vi "Teleop.vi"(0 "Call Context":T10) -> (6 "SubState 3":T1, 8 "SubState 4":T1, 9 "SubState 5":T9, 11 "Loop 3 Data":T5, 13 "Loop 4 Data":T4, 14 "SubState 0":T1=enum."driver control", 15 "Loop 1 Data":T7, 16 "Loop 0 Data":T8, 17 "SubState 1":T1, 18 "Loop 2 Data":T6, 19 "SubState 2":T1)   [LabVIEW 2013]
uses:
  typedefs/subStates.ctl
  <vilib>/Rock Robotics/WPI/DriverStation/WPI_DriverStationDerivedRobotMode.ctl
  typedefs/singleUseSubstate.ctl
  typedefs/Loop Datatypes/Loop 0 Datatype.ctl
  typedefs/Loop Datatypes/Loop 1 Datatype.ctl
  typedefs/Loop Datatypes/Loop 2 Datatype.ctl
  typedefs/Loop Datatypes/Loop 3 Datatype.ctl
  typedefs/Loop Datatypes/Loop 4 Datatype.ctl
  <vilib>/Rock Robotics/WPI/Joystick/WPI_JoystickDevRef.ctl
  <vilib>/Rock Robotics/WPI/Joystick/WPI_JoystickDeviceEnum.ctl
  typedefs/fg_typedef.ctl
  typedefs/vision enable.ctl
  <vilib>/Rock Robotics/WPI/Joystick/WPI_JoystickGetSetRefNum.vi
panel:
  out "prev lock state":T1
  out "JS3":T2
  out "Drive to DC":bool
  out "JS1":T2
  out "JS2":T2
  out "Exit Value":i32=-1
  # "Loop Data and Substates"
  # "Latch Loop"
  # "Drive Loop"
  # "Shooter Pneumatics Loop"
  # "Pickup/Passing Belts Loop"
  # "Pickup Arm Loop"
  # "Shifter Loop"
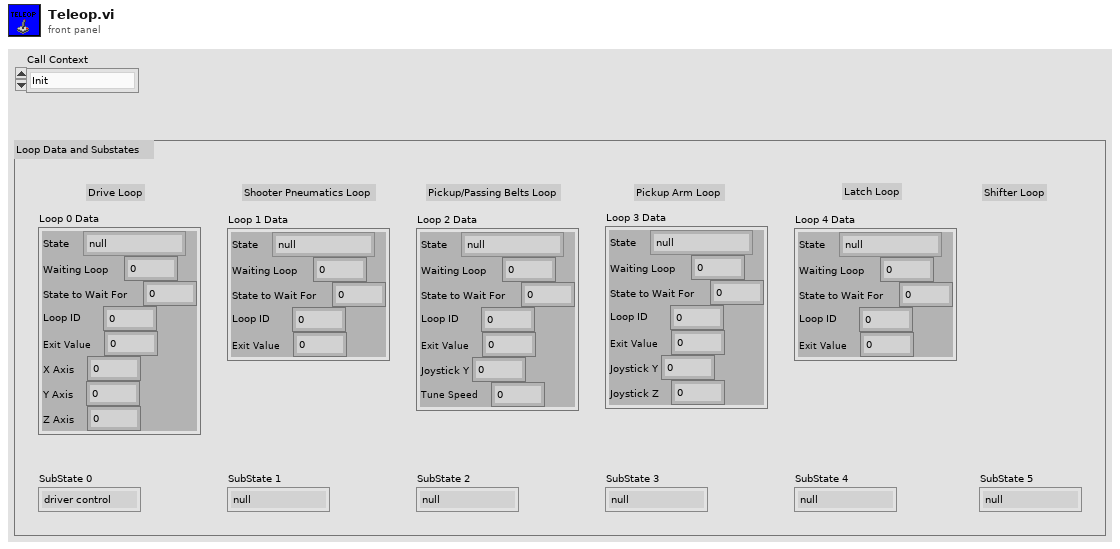
[diagram p1: front panel]
types:
  T1 = typedef "subStates.ctl" = enum16{"null", "wait", "driver control", "auto", "manual override", "hold position", "rotate", "pickup", "pass", "load", "goto shoot", "shoot", "cancel", "end"}
  T2 = typedef "WPI_JoystickDevRef.ctl" = cluster{"Device":T3}
  T3 = typedef "WPI_JoystickDeviceEnum.ctl" = enum16{"USB 1", "USB 2", "USB 3", "USB 4", "Kinect 1", "Kinect 2"}
  T4 = typedef "Loop 4 Datatype.ctl" = cluster{"State":T1, "Waiting Loop":i32, "State to Wait For":i32, "Loop ID":i32, "Exit Value":i32}
  T5 = typedef "Loop 3 Datatype.ctl" = cluster{"State":T1, "Waiting Loop":i32, "State to Wait For":i32, "Loop ID":i32, "Exit Value":i32, "Joystick Y":dbl, "Joystick Z":dbl}
  T6 = typedef "Loop 2 Datatype.ctl" = cluster{"State":T1, "Waiting Loop":i32, "State to Wait For":i32, "Loop ID":i32, "Exit Value":i32, "Joystick Y":dbl, "Tune Speed":dbl}
  T7 = typedef "Loop 1 Datatype.ctl" = cluster{"State":T1, "Waiting Loop":i32, "State to Wait For":i32, "Loop ID":i32, "Exit Value":i32}
  T8 = typedef "Loop 0 Datatype.ctl" = cluster{"State":T1, "Waiting Loop":i32, "State to Wait For":i32, "Loop ID":i32, "Exit Value":i32, "X Axis":dbl, "Y Axis":dbl, "Z Axis":dbl}
  T9 = typedef "singleUseSubstate.ctl" = enum16{"null", "wait", "shift high", "shift low"}
  T10 = typedef "WPI_DriverStationDerivedRobotMode.ctl" = enum16{"Init", "Execute", "Stop"}
  T11 = cluster{"axis 1 (x)":dbl, "axis 2 (y)":dbl, "axis 3 (throttle)":dbl, "axis 4":dbl, "axis 5":dbl, "axis 6":dbl}
  T12 = typedef "WPI_EncoderDevRef.ctl" = cluster{"DevStatus":errorcluster, "EncoderIndex":T13, "CounterIndex":T14, "DistancePerCount":dbl, "Decoding Type":T15}
  T13 = typedef "FPGA_EncoderIdx.ctl" = enum8{"Enc 0", "Enc 1", "Enc 2", "Enc 3", "Invalid"}
  T14 = typedef "FPGA_CounterCtrSystemIndex.ctl" = enum8{"Ctr 0", "Ctr 1", "Ctr 2", "Ctr 3", "Ctr 4", "Ctr 5", "Ctr 6", "Ctr 7", "Invalid"}
  T15 = typedef "WPI_EncoderType.ctl" = enum16{"1x", "2x", "4x"}
  T16 = typedef "vision enable.ctl" = enum16{"Enable", "Disable", "Stop"}
  T17 = typedef "fg_typedef.ctl" = enum16{"Get", "Set"}
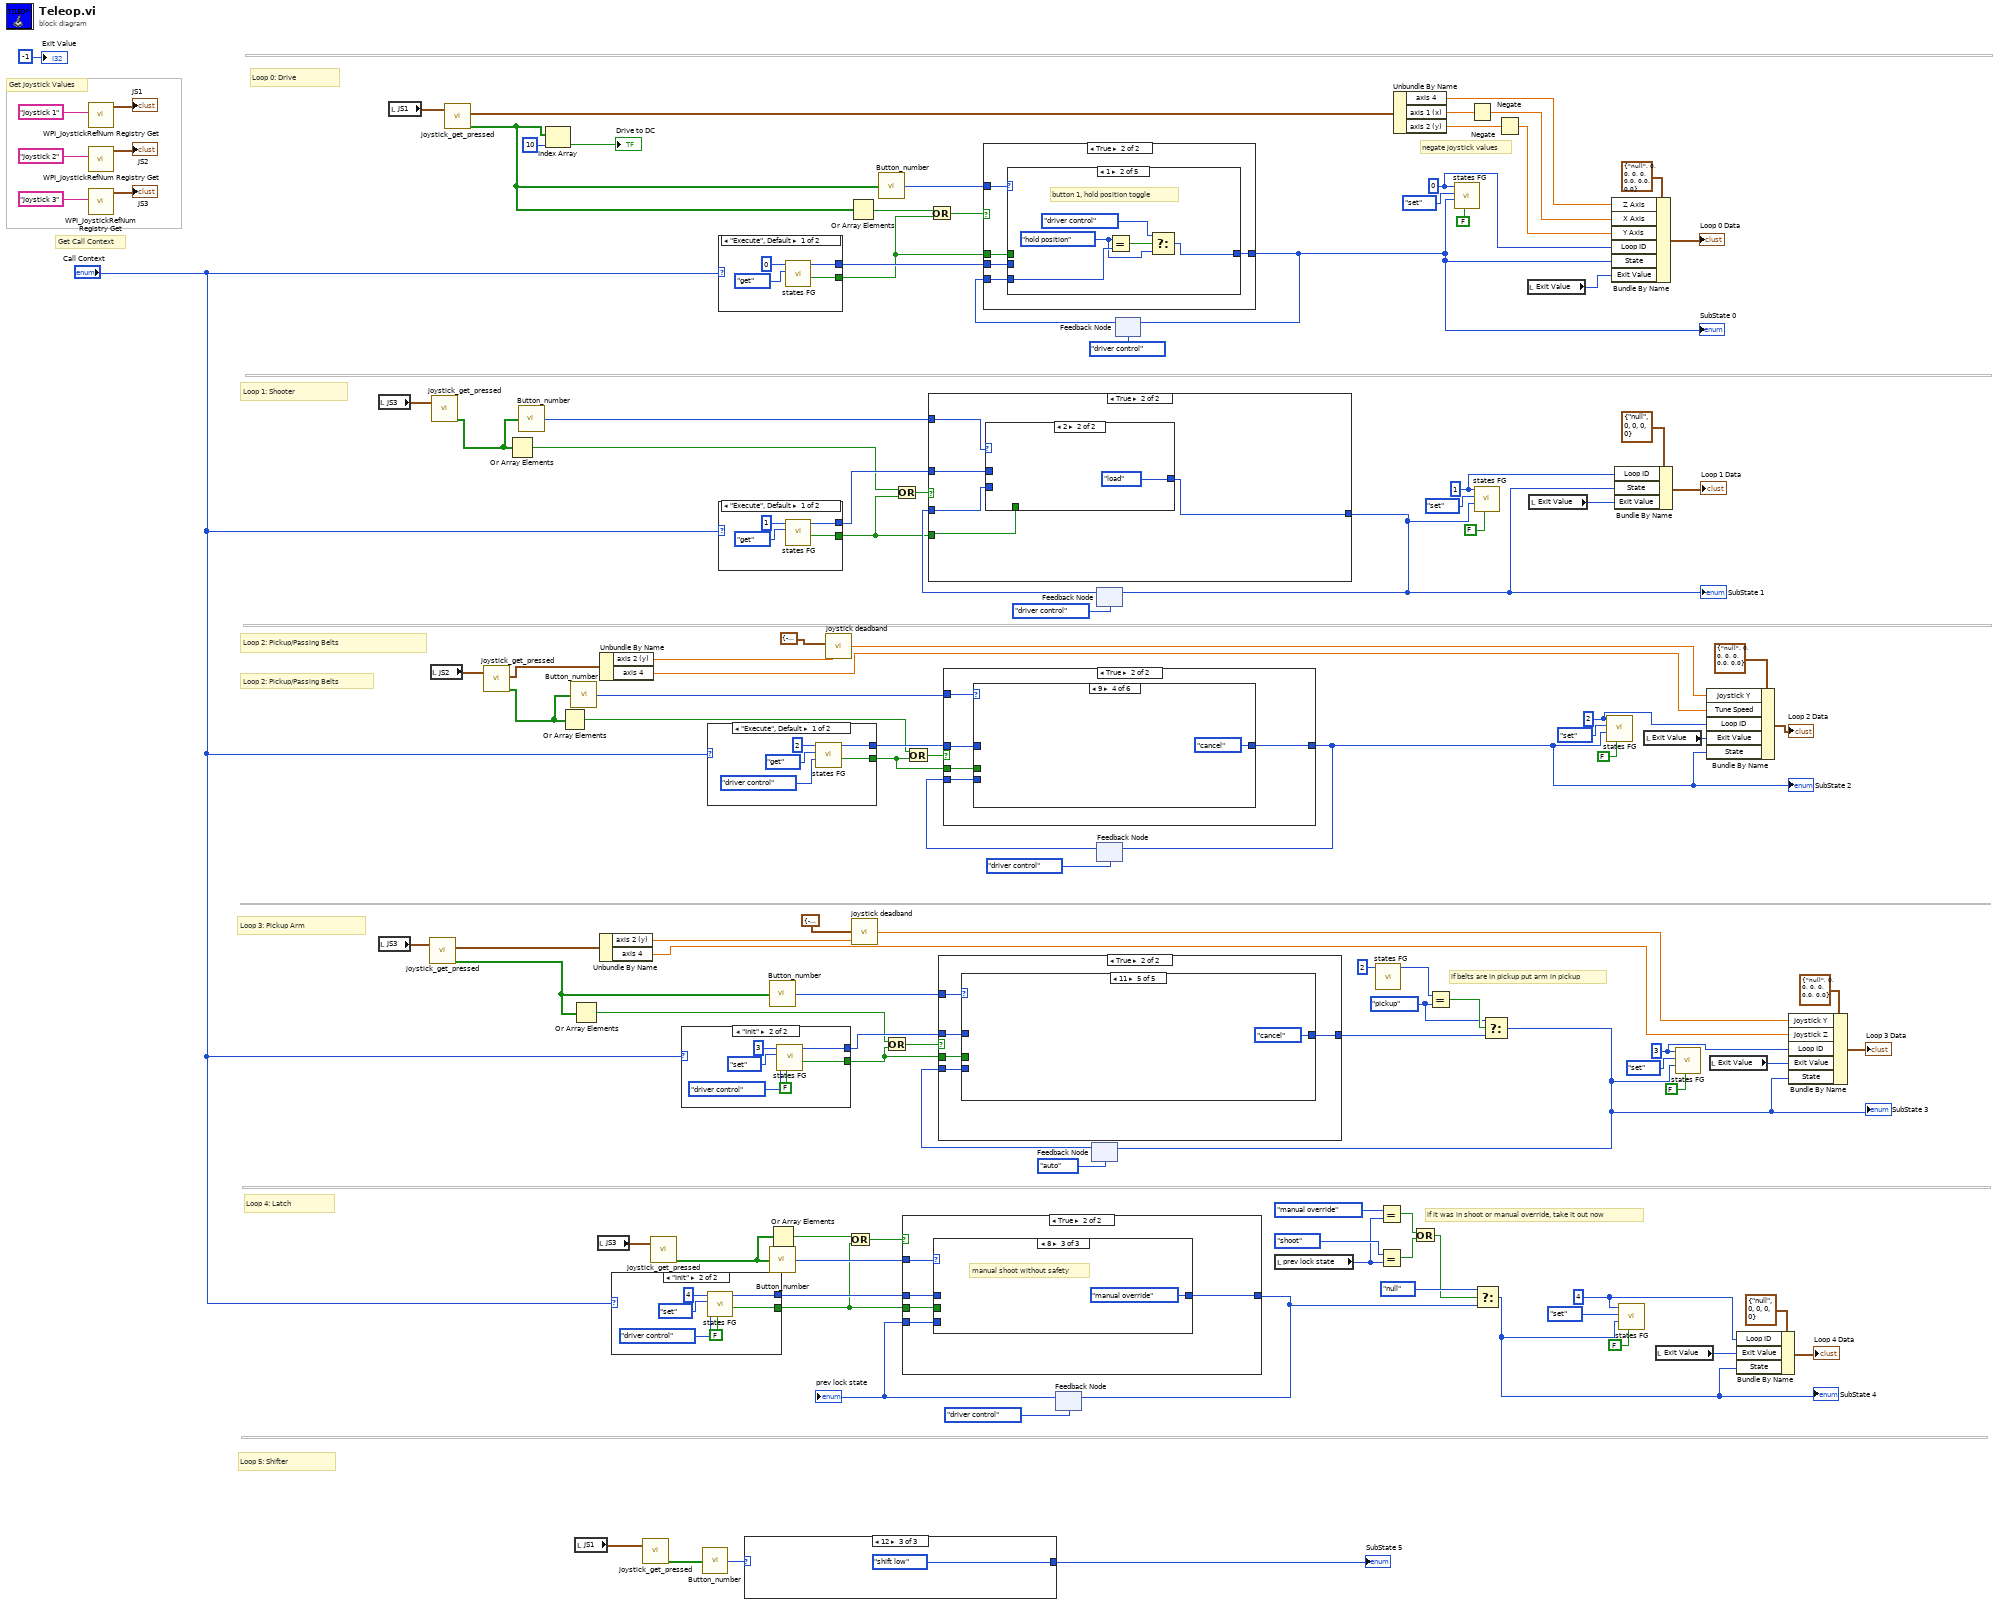
[diagram p0: block diagram]
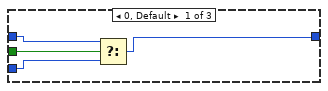
[diagram p3: hidden frame]
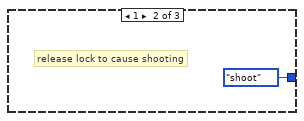
[diagram p4: hidden frame]
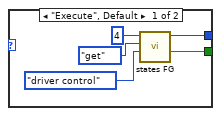
[diagram p5: hidden frame]
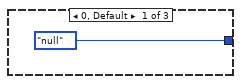
[diagram p6: hidden frame]
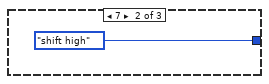
[diagram p7: hidden frame]
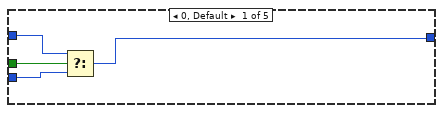
[diagram p9: hidden frame]
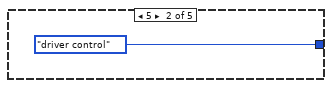
[diagram p10: hidden frame]
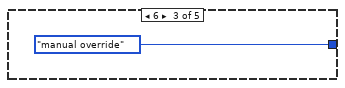
[diagram p11: hidden frame]
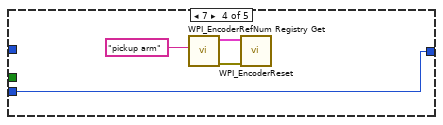
[diagram p12: hidden frame]
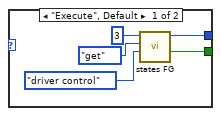
[diagram p13: hidden frame]
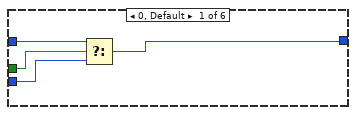
[diagram p15: hidden frame]
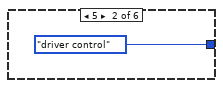
[diagram p16: hidden frame]
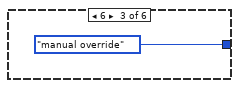
[diagram p17: hidden frame]
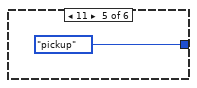
[diagram p18: hidden frame]
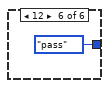
[diagram p19: hidden frame]
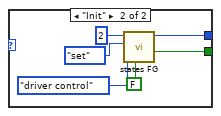
[diagram p20: hidden frame]
diagram:
  w10 = subStates."pickup" ("y")
  w29 = 4 ("Loop ID")
  w95 = 3 ("Loop ID")
  w96 = 2 ("Loop ID")
  w105 = 1 ("Loop ID")
  w107 = 0 ("Loop ID")
  # "if it was in shoot or manual override, take it out now"
  # "if belts are in pickup put arm in pickup"
  # "Loop 2: Pickup/Passing Belts"
  # "negate joystick values"
  # "Get Call Context"
  # "Get Joystick Values"
  # "Loop 4: Latch"
  # "Loop 3: Pickup Arm"
  # "Loop 5: Shifter"
  # "Loop 2: Pickup/Passing Belts"
  # "Loop 1: Shooter"
  # "Loop 0: Drive"
  n1 = call <vilib>:"WPI_JoystickRefNum Registry Get.vi"("refnum name"="Joystick 1") -> ("JoystickDevRef"=→"JS1":T2)  [unwired: 9 in, 1 out]
  n2 = call <vilib>:"WPI_JoystickRefNum Registry Get.vi"("refnum name"="Joystick 2") -> ("JoystickDevRef"=→"JS2":T2)  [unwired: 9 in, 1 out]
  n3 = call <vilib>:"WPI_JoystickRefNum Registry Get.vi"("refnum name"="Joystick 3") -> ("JoystickDevRef"=→"JS3":T2)  [unwired: 9 in, 1 out]
  n4 = local read "JS3"() -> (w72:T2)
  n5 = local read "JS3"() -> (w57:T2)
  n6 = local read "JS1"() -> (w73:T2)
  n7 = call "joystick_get_pressed.vi"("JoystickDevRef 2"=w57) -> ("Axes"=w61:T11, "Buttons Pressed?"=w38:bool[])  [unwired: 1 in, 2 out]
  n8 = local read "JS2"() -> (w45:T2)
  n9 = call "joystick_get_pressed.vi"("JoystickDevRef 2"=w72) -> ("Buttons Pressed?"=w40:bool[])  [unwired: 1 in, 3 out]
  n10 = call "joystick_get_pressed.vi"("JoystickDevRef 2"=w73) -> ("Axes"=w77:T11, "Buttons Pressed?"=w53:bool[])  [unwired: 1 in, 2 out]
  n11 = call "joystick_get_pressed.vi"("JoystickDevRef 2"=w45) -> ("Axes"=w26:T11, "Buttons Pressed?"=w27:bool[])  [unwired: 1 in, 2 out]
  n12 = Or Array Elements(Boolean array=w40) -> (logical OR=w64:bool)
  n13 = call "Button_number.vi"("Button Array"=w40) -> ("Button Pressed"=w66:i32)
  n14 = Index Array(array=w53, index=10) -> (element=→"Drive to DC":bool)
  n15 = Or Array Elements(Boolean array=w27) -> (logical OR=w44:bool)
  n16 = call "Button_number.vi"("Button Array"=w27) -> ("Button Pressed"=w43:i32)
  n17 = Or Array Elements(Boolean array=w38) -> (logical OR=w60:bool)
  n18 = local read "JS1"() -> (w48:T2)
  n19 = local read "JS3"() -> (w21:T2)
  n20 = Unbundle By Name(w61) -> ("axis 2 (y)"=w56:dbl, "axis 4"=w22:dbl)
  n21 = Unbundle By Name(w26) -> ("axis 2 (y)"=w37:dbl, "axis 4"=w24:dbl)
  n22 = case shown="\"Init\"" "Call Context" {
    tunnel: [w126 w132] -> w16
    tunnel: [w124 w129] -> w31
    frame "Execute", Default {
      n23 = call "states FG.vi"("subState in"=subStates."driver control", "menu (get)"=enum16{"set", "get"}."get", "Loop ID"=4) -> ("exit out"=w126:bool, "subState out"=w124:T1)  [unwired: 5 in, 2 out]
    }
    frame "Init" {
      n24 = call "states FG.vi"("exit in"=FALSE, "subState in"=subStates."driver control", "menu (get)"=enum16{"set", "get"}."set", "Loop ID"=4) -> ("exit out"=w132:bool, "subState out"=w129:T1)  [unwired: 4 in, 2 out]
    }
  }
  n25 = call "joystick_get_pressed.vi"("JoystickDevRef 2"=w48) -> ("Buttons Pressed?"=w50:bool[])  [unwired: 1 in, 3 out]
  n26 = call "joystick_get_pressed.vi"("JoystickDevRef 2"=w21) -> ("Buttons Pressed?"=w20:bool[])  [unwired: 1 in, 3 out]
  n27 = case shown="\"Init\"" "Call Context" {
    tunnel: [w137 w143] -> w58
    tunnel: [w135 w140] -> w93
    frame "Execute", Default {
      n28 = call "states FG.vi"("subState in"=subStates."driver control", "menu (get)"=enum16{"set", "get"}."get", "Loop ID"=3) -> ("exit out"=w137:bool, "subState out"=w135:T1)  [unwired: 5 in, 2 out]
    }
    frame "Init" {
      n29 = call "states FG.vi"("exit in"=FALSE, "subState in"=subStates."driver control", "menu (get)"=enum16{"set", "get"}."set", "Loop ID"=3) -> ("exit out"=w143:bool, "subState out"=w140:T1)  [unwired: 4 in, 2 out]
    }
  }
  n30 = call "Button_number.vi"("Button Array"=w50) -> ("Button Pressed"=w49:i32)
  n31 = case shown="\"Execute\", Default" "Call Context" {
    tunnel: [w148 w154] -> w63
    tunnel: [w146 w151] -> w112
    frame "Execute", Default {
      n32 = call "states FG.vi"("subState in"=subStates."driver control", "menu (get)"=enum16{"set", "get"}."get", "Loop ID"=2) -> ("exit out"=w148:bool, "subState out"=w146:T1)  [unwired: 5 in, 2 out]
    }
    frame "Init" {
      n33 = call "states FG.vi"("exit in"=FALSE, "subState in"=subStates."driver control", "menu (get)"=enum16{"set", "get"}."set", "Loop ID"=2) -> ("exit out"=w154:bool, "subState out"=w151:T1)  [unwired: 4 in, 2 out]
    }
  }
  n34 = case shown="\"Execute\", Default" "Call Context" {
    tunnel: [w158 w163] -> w70
    tunnel: [w157 w161] -> w110
    frame "Execute", Default {
      n35 = call "states FG.vi"("menu (get)"=enum16{"set", "get"}."get", "Loop ID"=0) -> ("exit out"=w158:bool, "subState out"=w157:T1)  [unwired: 6 in, 2 out]
    }
    frame "Init" {
      n36 = call "states FG.vi"("exit in"=FALSE, "menu (get)"=enum16{"set", "get"}."set", "Loop ID"=0) -> ("exit out"=w163:bool, "subState out"=w161:T1)  [unwired: 5 in, 2 out]
    }
  }
  n37 = case shown="\"Execute\", Default" "Call Context" {
    tunnel: [w167 w172] -> w67
    tunnel: [w166 w170] -> w109
    frame "Execute", Default {
      n38 = call "states FG.vi"("menu (get)"=enum16{"set", "get"}."get", "Loop ID"=1) -> ("exit out"=w167:bool, "subState out"=w166:T1)  [unwired: 6 in, 2 out]
    }
    frame "Init" {
      n39 = call "states FG.vi"("exit in"=FALSE, "menu (get)"=enum16{"set", "get"}."set", "Loop ID"=1) -> ("exit out"=w172:bool, "subState out"=w170:T1)  [unwired: 5 in, 2 out]
    }
  }
  n40 = case shown="12" w49 {
    tunnel: [singleUseSubstate."null" ("Enum") singleUseSubstate."shift high" ("Enum") singleUseSubstate."shift low" ("Enum")] -> w85
    frame 0, Default {
    }
    frame 7 {
    }
    frame 12 {
    }
  }
  "SubState 5" <- w85
  n41 = call "Button_number.vi"("Button Array"=w38) -> ("Button Pressed"=w59:i32)
  n42 = call "Button_number.vi"("Button Array"=w20) -> ("Button Pressed"=w17:i32)
  n43 = Or Array Elements(Boolean array=w20) -> (logical OR=w19:bool)
  n44 = call "joystick deadband.vi"("Joystick In"=w37, "Deadband Range"=cluster{"Deadband Min":dbl, "Deadband Max":dbl} {"Deadband Min"=-0.05, "Deadband Max"=0.05}) -> ("Joystick Out"=w25:dbl)  [unwired: 4 in]
  n45 = Or(x=w19, y=w16) -> (x .or. y?=w18:bool)
  n46 = Or Array Elements(Boolean array=w53) -> (logical OR=w71:bool)
  n47 = call "joystick deadband.vi"("Joystick In"=w56, "Deadband Range"=cluster{"Deadband Min":dbl, "Deadband Max":dbl} {"Deadband Min"=-0.05, "Deadband Max"=0.05}) -> ("Joystick Out"=w23:dbl)  [unwired: 4 in]
  n48 = call "Button_number.vi"("Button Array"=w53) -> ("Button Pressed"=w76:i32)
  n49 = Or(x=w60, y=w58) -> (x .or. y?=w62:bool)
  n50 = Or(x=w64, y=w67) -> (x .or. y?=w68:bool)
  n51 = Or(x=w44, y=w63) -> (x .or. y?=w65:bool)
  n52 = Or(x=w71, y=w70) -> (x .or. y?=w69:bool)
  n53 = feedback #1(subStates."driver control" ("Drive SubState")) -> (w34:T1)
  "prev lock state" <- w34
  n54 = case shown="True" w18 {
    tunnel: w34 -> [w178 w180]
    tunnel: [w178 w179] -> w8
    tunnel: w31 -> [_ w182]
    tunnel: w17 -> [_ w183]
    tunnel: w16 -> [_ w181]
    frame False {
      # "*yawn* nothing to do...wire through the previous state"
    }
    frame True {
      n55 = case shown="8" w183 {
        tunnel: w182 -> [w186 _ _]
        tunnel: w181 -> [w187 _ _]
        tunnel: w180 -> [w185 _ _]
        tunnel: [w184 subStates."shoot" ("Drive SubState") subStates."manual override" ("Drive SubState")] -> w179
        frame 0, Default {
          n56 = Select(t=w186, s=w187, f=w185) -> (s? t:f=w184:T1)
        }
        frame 1 {
          # "release lock to cause shooting"
        }
        frame 8 {
          # "manual shoot without safety"
        }
      }
    }
  }
  n57 = feedback-in #1(w8) -> ()
  n58 = feedback #2(subStates."auto" ("Drive SubState")) -> (w90:T1)
  n59 = case shown="True" w62 {
    tunnel: w90 -> [w190 w191]
    tunnel: [w190 w192] -> w13
    tunnel: w93 -> [_ w193]
    tunnel: w59 -> [_ w195]
    tunnel: w58 -> [_ w194]
    frame False {
      # "boring drivers, not pressing anything...wire through the previous state"
    }
    frame True {
      n60 = case shown="11" w195 {
        tunnel: w194 -> [w199 _ _ _ _]
        tunnel: w191 -> [w198 _ _ w205 _]
        tunnel: w193 -> [w197 _ _ _ _]
        tunnel: [w196 subStates."driver control" ("Drive SubState") subStates."manual override" ("Drive SubState") w205 subStates."cancel" ("Drive SubState")] -> w192
        frame 0, Default {
          n61 = Select(t=w197, s=w199, f=w198) -> (s? t:f=w196:T1)
        }
        frame 5 {
        }
        frame 6 {
        }
        frame 7 {
          n62 = call <vilib>:"WPI_EncoderRefNum Registry Get.vi"("refnum name"="pickup arm") -> ("error out"=w203:errorcluster, "EncoderDevRef"=w202:T12)  [unwired: 9 in]
          n63 = call <vilib>:"WPI_EncoderReset.vi"("error in (no error)"=w203, "EncoderDevRef"=w202) -> ()  [unwired: 8 in, 2 out]
        }
        frame 11 {
        }
      }
    }
  }
  n64 = feedback #3(subStates."driver control" ("Drive SubState")) -> (w111:T1)
  n65 = case shown="True" w68 {
    tunnel: w111 -> [w207 w211]
    tunnel: [w207 w208] -> w78
    tunnel: w109 -> [_ w212]
    tunnel: w66 -> [_ w210]
    tunnel: w67 -> [_ w209]
    frame False {
      # "nothing pressed here, move along (wire through the previous state)"
    }
    frame True {
      n66 = case shown="2" w210 {
        tunnel: w212 -> [w215 _]
        tunnel: w211 -> [w214 _]
        tunnel: [w213 subStates."load" ("Drive SubState")] -> w208
        tunnel: w209 -> [w216 _]
        frame 0, Default {
          n67 = Select(t=w215, s=w216, f=w214) -> (s? t:f=w213:T1)
        }
        frame 2 {
        }
      }
    }
  }
  "SubState 1" <- w78
  n68 = feedback-in #3(w78) -> ()
  n69 = feedback #4(subStates."driver control" ("Drive SubState")) -> (w115:T1)
  n70 = case shown="True" w65 {
    tunnel: w115 -> [w218 w220]
    tunnel: [w218 w219] -> w36
    tunnel: w112 -> [_ w221]
    tunnel: w43 -> [_ w223]
    tunnel: w63 -> [_ w222]
    frame False {
      # "nothing pressed here, move along obviously and wire through the previous state"
    }
    frame True {
      n71 = case shown="9" w223 {
        tunnel: w222 -> [w227 _ _ _ _ _]
        tunnel: w221 -> [w226 _ _ _ _ _]
        tunnel: w220 -> [w225 _ _ _ _ _]
        tunnel: [w224 subStates."driver control" ("Drive SubState") subStates."manual override" ("Drive SubState") subStates."cancel" ("Drive SubState") subStates."pickup" ("Drive SubState") subStates."pass" ("Drive SubState")] -> w219
        frame 0, Default {
          n72 = Select(t=w226, s=w227, f=w225) -> (s? t:f=w224:T1)
        }
        frame 5 {
        }
        frame 6 {
        }
        frame 9 {
        }
        frame 11 {
        }
        frame 12 {
        }
      }
    }
  }
  "SubState 2" <- w36
  n73 = feedback-in #4(w36) -> ()
  n74 = feedback #5(subStates."driver control" ("Drive SubState")) -> (w117:T1)
  n75 = case shown="True" w69 {
    tunnel: w117 -> [w233 w235]
    tunnel: [w233 w234] -> w47
    tunnel: w110 -> [_ w236]
    tunnel: w76 -> [_ w238]
    tunnel: w70 -> [_ w237]
    frame False {
      # "keep current state, no change necessary"
    }
    frame True {
      n76 = case shown="1" w238 {
        tunnel: w237 -> [w242 _ _ _ _]
        tunnel: w236 -> [w241 _ _ _ _]
        tunnel: w235 -> [w240 w247 w248 _ _]
        tunnel: [w239 w243 w248 subStates."goto shoot" ("Drive SubState") subStates."driver control" ("Drive SubState")] -> w234
        frame 0, Default {
          n77 = Select(t=w241, s=w242, f=w240) -> (s? t:f=w239:T1)
        }
        frame 1 {
          w244 = subStates."hold position" ("x")
          # "button 1, hold position toggle"
          n78 = Equal?(x=w244, y=w247) -> (x = y?=w246:bool)
          n79 = Select(t=subStates."driver control" ("Drive SubState"), s=w246, f=w244) -> (s? t:f=w243:T1)
        }
        frame 8 {
          w251 = vision_enable."Enable" ("y")
          # "toggle vision"
          n80 = call "vision_fg.vi"("Menu"=fg_typedef."Get") -> ("State Out"=w253:T16)  [unwired: 2 in, 1 out]
          n81 = Equal?(x=w253, y=w251) -> (x = y?=w252:bool)
          n82 = Select(t=vision_enable."Disable" ("y"), s=w252, f=w251) -> (s? t:f=w249:T16)
          n83 = call "vision_fg.vi"("Action"=w249, "Menu"=fg_typedef."Set") -> ()  [unwired: 1 in, 2 out]
        }
        frame 9 {
          # "go to shoot location"
          n84 = call "vision_fg.vi"("Action"=vision_enable."Enable", "Menu"=fg_typedef."Set") -> ()  [unwired: 1 in, 2 out]
        }
        frame 11 {
          # "put robot drive in driver control"
          n85 = call "vision_fg.vi"("Action"=vision_enable."Disable", "Menu"=fg_typedef."Set") -> ()  [unwired: 1 in, 2 out]
        }
      }
    }
  }
  "SubState 0" <- w47
  n86 = feedback-in #5(w47) -> ()
  n87 = local read "prev lock state"() -> (w5:T1)
  n88 = call "states FG.vi"("Loop ID"=2) -> ("subState out"=w14:T1)  [unwired: 7 in, 3 out]
  n89 = Equal?(x=subStates."manual override", y=w5) -> (x = y?=w2:bool)
  n90 = Equal?(x=subStates."shoot", y=w5) -> (x = y?=w3:bool)
  n91 = Unbundle By Name(w77) -> ("axis 4"=w54:dbl, "axis 1 (x)"=w82:dbl, "axis 2 (y)"=w81:dbl)
  n92 = Or(x=w2, y=w3) -> (x .or. y?=w1:bool)
  n93 = Equal?(x=w14, y=w10) -> (x = y?=w11:bool)
  n94 = call "states FG.vi"("exit in"=FALSE, "subState in"=w47, "menu (get)"=enum16{"set", "get"}."set", "Loop ID"=w107) -> ()  [unwired: 4 in, 4 out]
  n95 = Negate(x=w82) -> (-x=w80:dbl)
  n96 = call "states FG.vi"("exit in"=FALSE, "subState in"=w78, "menu (get)"=enum16{"set", "get"}."set", "Loop ID"=w105) -> ()  [unwired: 4 in, 4 out]
  n97 = Select(t=subStates."null", s=w1, f=w8) -> (s? t:f=w7:T1)
  "SubState 4" <- w7
  n98 = Select(t=w10, s=w11, f=w13) -> (s? t:f=w12:T1)
  "SubState 3" <- w12
  n99 = feedback-in #2(w12) -> ()
  n100 = Negate(x=w81) -> (-x=w79:dbl)
  n101 = local read "Exit Value"() -> (w103:i32)
  n102 = local read "Exit Value"() -> (w102:i32)
  n103 = call "states FG.vi"("exit in"=FALSE, "subState in"=w36, "menu (get)"=enum16{"set", "get"}."set", "Loop ID"=w96) -> ()  [unwired: 4 in, 4 out]
  n104 = Bundle By Name(cluster=T8 {"State"=enum."null", "Waiting Loop"=0, "State to Wait For"=0, "Loop ID"=0, "Exit Value"=0, "X Axis"=0.0, "Y Axis"=0.0, "Z Axis"=0.0} ("Cluster"), "Z Axis"=w54, "X Axis"=w80, "Y Axis"=w79, "Loop ID"=w107, "State"=w47, "Exit Value"=w103) -> (→"Loop 0 Data":T8)
  n105 = Bundle By Name(cluster=T7 {"State"=enum."null", "Waiting Loop"=0, "State to Wait For"=0, "Loop ID"=0, "Exit Value"=0} ("Cluster"), "Loop ID"=w105, "State"=w78, "Exit Value"=w102) -> (→"Loop 1 Data":T7)
  n106 = call "states FG.vi"("exit in"=FALSE, "subState in"=w7, "menu (get)"=enum16{"set", "get"}."set", "Loop ID"=w29) -> ()  [unwired: 4 in, 4 out]
  n107 = local read "Exit Value"() -> (w97:i32)
  n108 = local read "Exit Value"() -> (w30:i32)
  n109 = call "states FG.vi"("exit in"=FALSE, "subState in"=w12, "menu (get)"=enum16{"set", "get"}."set", "Loop ID"=w95) -> ()  [unwired: 4 in, 4 out]
  n110 = Bundle By Name(cluster=T6 {"State"=enum."null", "Waiting Loop"=0, "State to Wait For"=0, "Loop ID"=0, "Exit Value"=0, "Joystick Y"=0.0, "Tune Speed"=0.0} ("Loop 2 Data"), "Joystick Y"=w25, "Tune Speed"=w24, "Loop ID"=w96, "Exit Value"=w97, "State"=w36) -> (→"Loop 2 Data":T6)
  n111 = local read "Exit Value"() -> (w94:i32)
  n112 = Bundle By Name(cluster=T4 {"State"=enum."null", "Waiting Loop"=0, "State to Wait For"=0, "Loop ID"=0, "Exit Value"=0} ("Loop 4 Data"), "Loop ID"=w29, "Exit Value"=w30, "State"=w7) -> (→"Loop 4 Data":T4)
  n113 = Bundle By Name(cluster=T5 {"State"=enum."null", "Waiting Loop"=0, "State to Wait For"=0, "Loop ID"=0, "Exit Value"=0, "Joystick Y"=0.0, "Joystick Z"=0.0} ("Loop 3 Data"), "Joystick Y"=w23, "Joystick Z"=w22, "Loop ID"=w95, "Exit Value"=w94, "State"=w12) -> (→"Loop 3 Data":T5)
  "Exit Value" <- -1 ("Exit Value")
